vi "append_to_log.vi"(8 "error in":errorcluster, 11 "string":string) -> (0 "error out":errorcluster)   [LabVIEW 2013]
uses:
  Experiment/Globals.vi
  Experiment/Experiment.lvclass
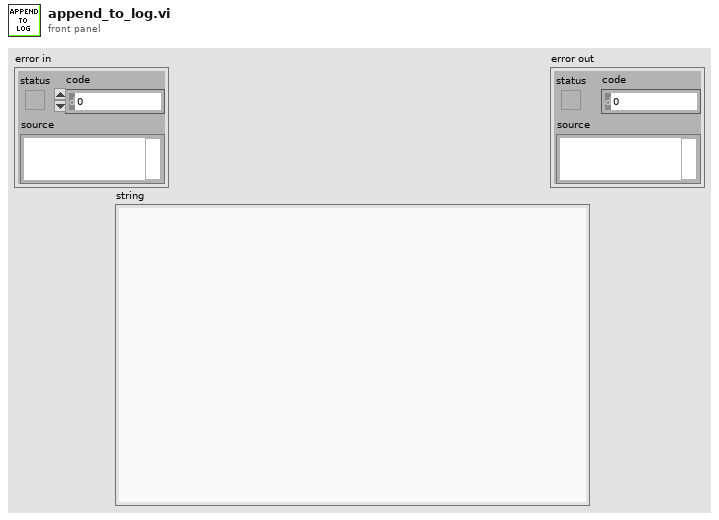
[diagram p1: front panel]
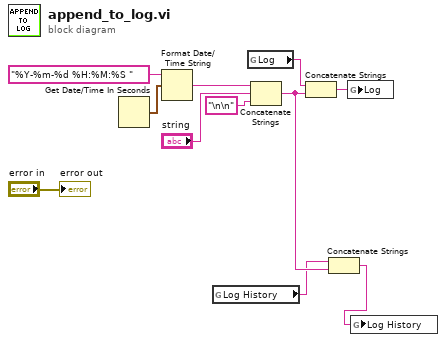
[diagram p0: block diagram]
diagram:
  n1 = Get Date/Time In Seconds() -> (seconds since 1Jan1904=w11:timestamp)
  n2 = Format Date/Time String(time format string (%c)="%Y-%m-%d %H:%M:%S ", seconds (now)=w11) -> (date/time string=w9:string)  [unwired: 1 in]
  n3 = global read "Globals.vi" "Log History"() -> (w2:string)
  n4 = global read "Globals.vi" "Log"() -> (w4:string)
  n5 = Concatenate Strings(w9, "string", "\n\n" ("string")) -> (w3:string)
  n6 = Concatenate Strings(w4, w3) -> (w5:string)
  n7 = Concatenate Strings(w2, w3) -> (w1:string)
  n8 = global write "Globals.vi" "Log"(w5) -> ()
  n9 = global write "Globals.vi" "Log History"(w1) -> ()
  "error out" <- "error in"
